vi "Round.vi"(0 "x":dbl) -> (4 "x rounded":dbl, 6 "x rounded to nearest half down":dbl, 8 "x rounded to nearest half up":dbl)   [LabVIEW 2012, in "ni579x Synchronization v1 Host.lvlib"]
uses:
  <instrlib>/ni579x/Synchronization/v1/Host/ni579x Synchronization v1 Host.lvlib
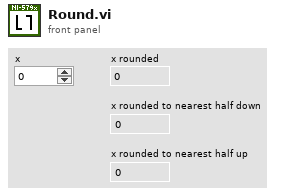
[diagram p1: front panel]
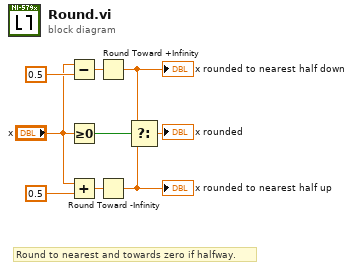
[diagram p0: block diagram]
diagram:
  # "Round to nearest and towards zero if halfway."
  n1 = Subtract(x="x", y=0.5) -> (x-y=w4:dbl)
  n2 = Greater Or Equal To 0?(x="x") -> (x >= 0?=w8:bool)
  n3 = Add(x="x", y=0.5) -> (x+y=w6:dbl)
  n4 = Round Toward +Infinity(x=w4) -> (ceil(x): smallest int >= x=w1:dbl)
  "x rounded to nearest half down" <- w1
  n5 = Round Toward -Infinity(1:w6) -> (0:w3:dbl)
  "x rounded to nearest half up" <- w3
  n6 = Select(t=w1, s=w8, f=w3) -> (s? t:f=→"x rounded":dbl)
